vi "ConfigWindow.vi"(8 "error in":errorcluster) -> (0 "error out":errorcluster, 3 "COM Bluegiga out":refnum<visa-resource-name>, 4 "Connection Status":T1={"MAC Address"="", "cnx handle"=0, "cnx flags"=0, "Address Type"=0, "Connection Interval (ms)"=125, "Timeout(ms)"=125, "Latency"=125, "bonding handle"=0} {"Address Type" items=["Public", "Random"]})   [LabVIEW 2015]
uses:
  <vilib>/BLE/type_def/connection_status_bundle.ctl
  <vilib>/BLE/type_def/address_type.ctl
panel:
  in  "Save to Database":bool=TRUE
  in  "CONNECT":bool caption="Power"
  out "Choosen adress":string caption="String"
  out "Tab":string[][](array[string]) caption="Donge info"
  in  "SCAN":bool caption="Search"
  out "Donge info":string caption="String"
  in  "BLE Dongle VISA":refnum<visa-resource-name>
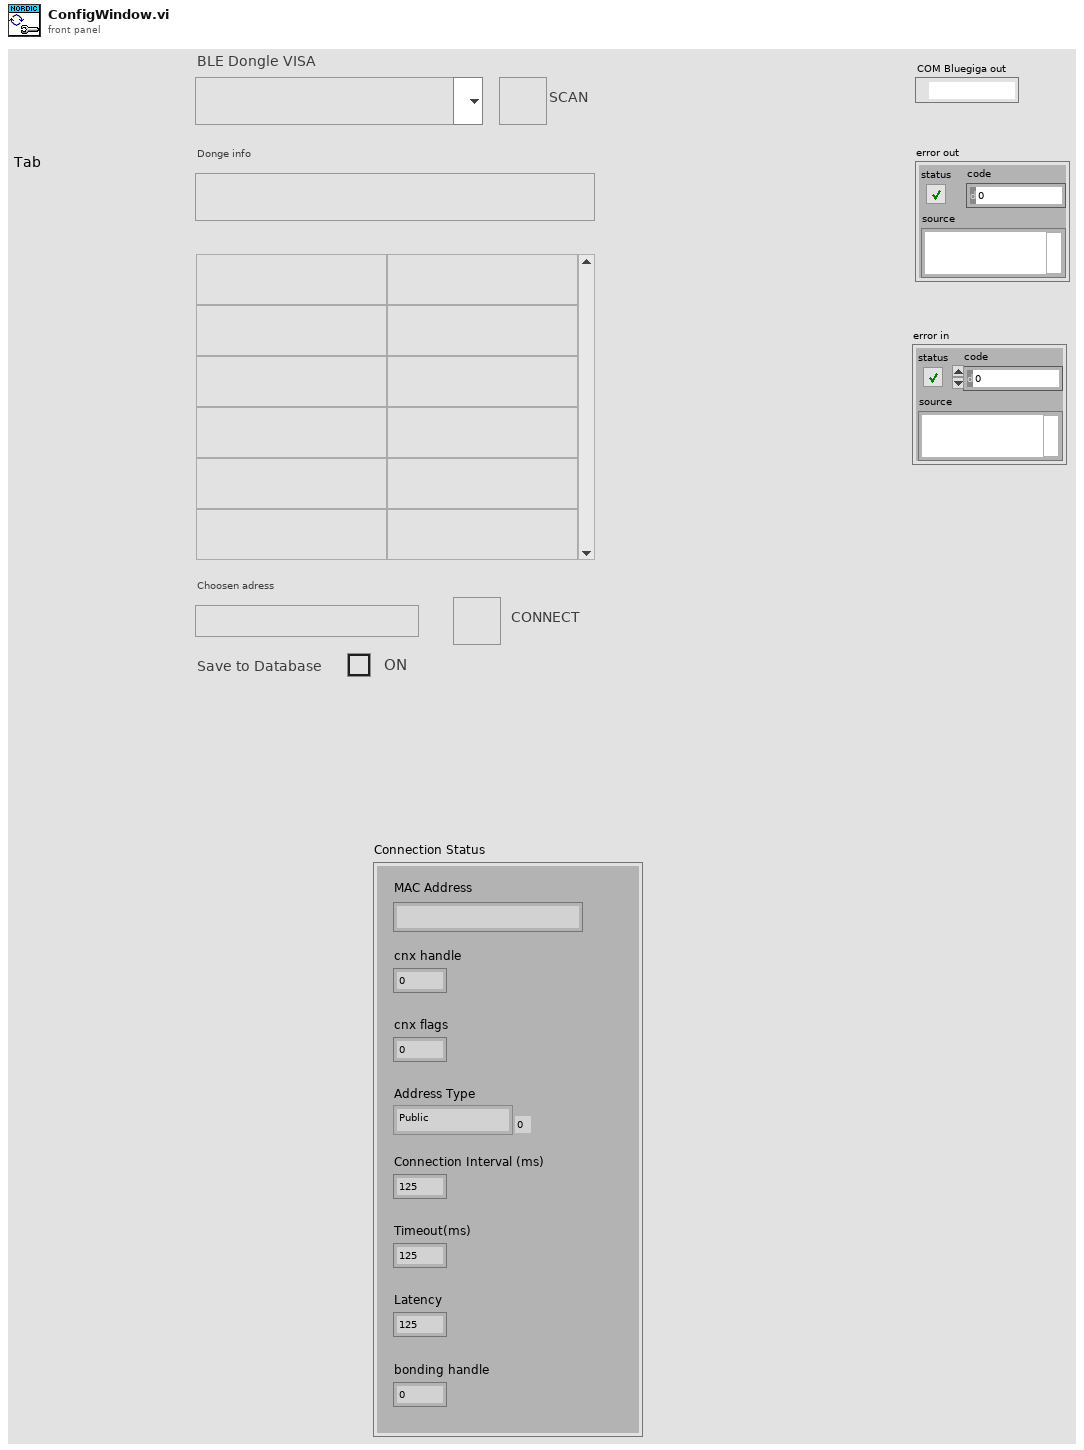
[diagram p1: front panel]
types:
  T1 = typedef "connection_status_bundle.ctl" = cluster{"MAC Address":string, "cnx handle":u8, "cnx flags":u8, "Address Type":T2, "Connection Interval (ms)":u16, "Timeout(ms)":u16, "Latency":u16, "bonding handle":u8}
  T2 = typedef "address_type.ctl" = u8
  T3 = enum8{"Enabled", "Disabled", "Disabled and Grayed Out"}
  T4 = typedef "LVPoint32TypeDef.ctl" = cluster{"Horizontal":i32, "Vertical":i32}
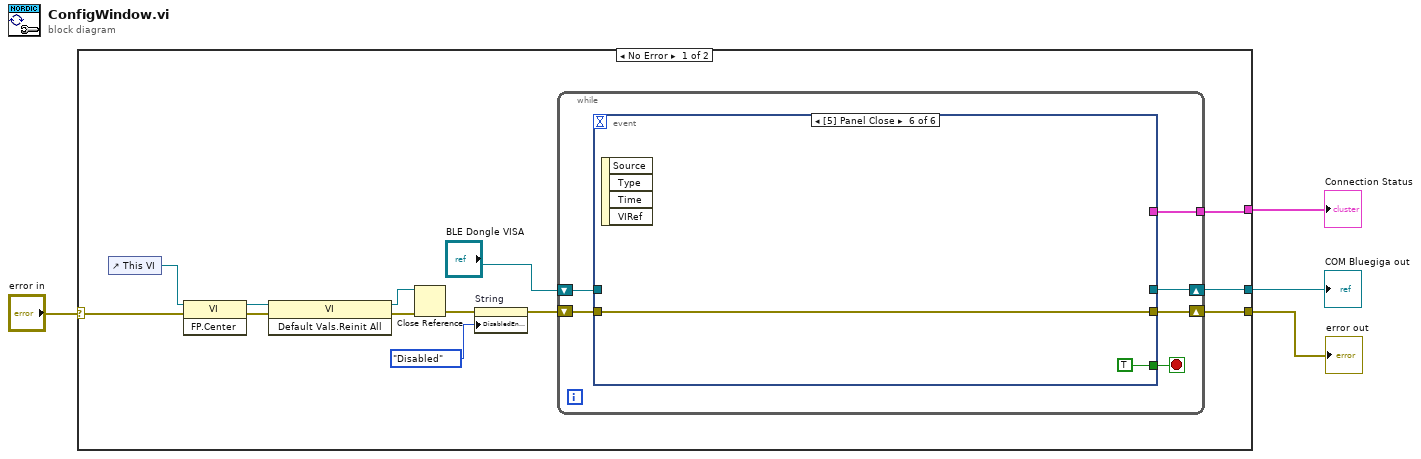
[diagram p0: block diagram]
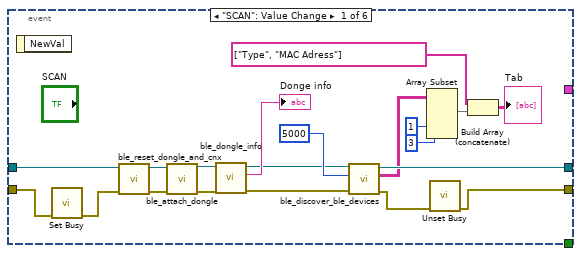
[diagram p2: hidden frame]
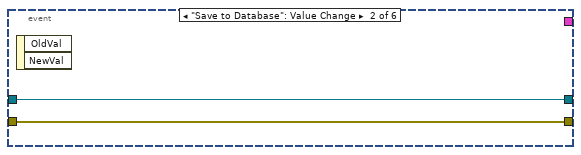
[diagram p3: hidden frame]
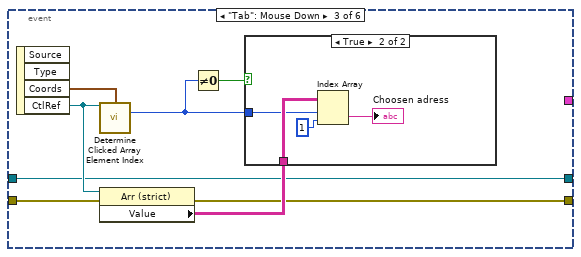
[diagram p4: hidden frame]
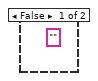
[diagram p5: hidden frame]
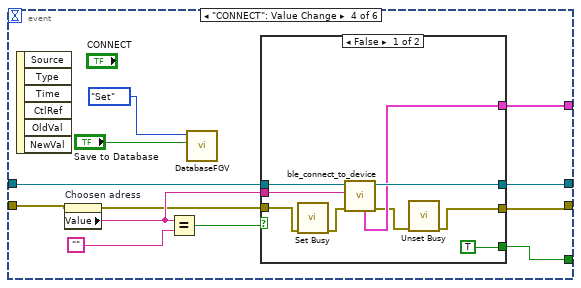
[diagram p6: hidden frame]
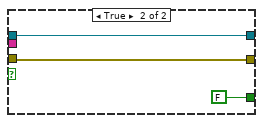
[diagram p7: hidden frame]
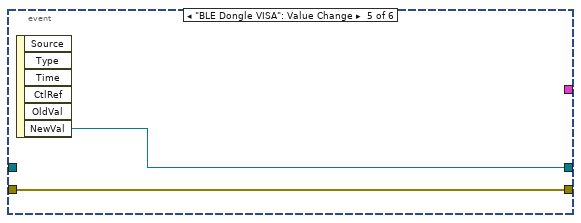
[diagram p8: hidden frame]
diagram:
  n1 = case shown="No Error" "error in" {
    selector: "error in" -> [w9 w86]
    tunnel: [w15 _] -> w4
    tunnel: [w14 w86] -> w3
    tunnel: [w5 _] -> w1
    frame No Error {
      n2 = control-ref of="This VI"() -> (w8:refnum<vi>)
      n3 = invoke class="VI" method="FP.Center"(reference=w8, error in=w9) -> (reference out=w7:refnum<vi>, error out=w6:errorcluster)  [unwired: 1 in, 1 out]
      n4 = invoke class="VI" method="Default Vals.Reinit All"(reference=w7, error in=w6) -> (reference out=w11:refnum<vi>, error out=w12:errorcluster)  [unwired: 1 in, 1 out]
      n5 = Close Reference(reference=w11, error in (no error)=w12) -> (error out=w10:errorcluster)
      n6 = property on="String" class="Str"(error in=w10, "DisabledEnum"=T3."Disabled" ("Disabled")) -> (error out=w13:errorcluster)  [unwired: 1 in, 1 out]
      n7 = while {
        shift-right: [w20] -> w14
        shift-left: w13 -> [w22]
        shift-right: [w19] -> w15
        shift-left: "BLE Dongle VISA" -> [w23]
        tunnel: [w18] -> w5
        stop <- w21 stop-if-true
        n8 = event shown="[5] Panel Close" {
          selector: _ -> [_ _ _ _ _ _]
          dyn-events: _ -> [_ _ _ _ _ _]
          timeout: _ -> [_ _ _ _ _ _]
          tunnel: w23 -> [w40 w44 w46 w63 _ _]
          tunnel: w22 -> [w37 w45 w51 w66 w82 w84]
          tunnel: [w31 w44 w46 w61 w83 _] -> w19
          tunnel: [_ _ _ w67 _ TRUE] -> w21
          tunnel: [w27 w45 w49 w62 w82 w84] -> w20
          tunnel: [_ _ _ w60 _ _] -> w18
          event "SCAN": Value Change {
            n9 = event-data() -> ()  [unwired: 1 in, 1 out]
            n10 = call <vilib>:"Set Busy.vi"("error in (no error)"=w37) -> ("error out"=w36:errorcluster)  [unwired: 9 in, 1 out]
            n11 = call <vilib>:"ble_reset_dongle_and_cnx.vi"("error in (no error)"=w36, "COM Bluegiga in"=w40) -> ("error out"=w39:errorcluster, "COM Bluegiga out"=w42:refnum<visa-resource-name>)  [unwired: 8 in]
            n12 = call <vilib>:"ble_attach_dongle.vi"("error in (no error)"=w39, "COM Bluegiga in"=w42) -> ("error out"=w38:errorcluster, "COM Bluegiga out"=w41:refnum<visa-resource-name>)  [unwired: 8 in]
            n13 = call <vilib>:"ble_dongle_info.vi"("error in (no error)"=w38, "COM Bluegiga in"=w41) -> ("error out"=w34:errorcluster, "info"=→"Donge info":string, "COM Bluegiga out"=w33:refnum<visa-resource-name>)  [unwired: 7 in]
            n14 = call <vilib>:"ble_discover_ble_devices.vi"("error in (no error)"=w34, "Scan Duration (10000ms)"=u32 5000, "COM Bluegiga in"=w33) -> ("error out"=w32:errorcluster, "Devices"=w30:string[][], "COM Bluegiga out"=w31:refnum<visa-resource-name>)  [unwired: 6 in]
            n15 = Array Subset(array=w30, index (col)=1 ("index"), length (col)=3 ("index")) -> (w25:string[][])  [unwired: 2 in]
            n16 = call <vilib>:"Unset Busy.vi"("error in (no error)"=w32) -> ("error out"=w27:errorcluster)  [unwired: 10 in]
            n17 = Build Array (concatenate)(string[] ["Type", "MAC Adress"] ("element"), w25) -> (→"Tab":string[][])
          }
          event "Save to Database": Value Change {
            n18 = event-data() -> ()  [unwired: 1 in, 2 out]
          }
          event "Tab": Mouse Down {
            n19 = event-data() -> ("Coords"=w52:T4, "CtlRef"=w50:refnum<vi>)  [unwired: 1 in, 2 out]
            n20 = call "Determine Clicked Array Element Index.vi"("reference"=w50, "Coords of Click"=w52) -> ("Clicked Row"=w47:i32)  [unwired: 8 in, 5 out]
            n21 = property class="Arr (strict)"(reference=w50, error in=w51) -> (error out=w49:errorcluster, "Value"=w53:string[][])  [unwired: 1 out]
            n22 = Not Equal To 0?(x=w47) -> (x != 0?=w48:bool)
            n23 = case shown="True" w48 {
              tunnel: w53 -> [_ w57]
              tunnel: w47 -> [_ w55]
              frame False {
                (unwired) "" ("String")
              }
              frame True {
                n24 = Index Array(array=w57, index (row)=w55, index (col)=1 ("disabled index (col)")) -> (element=→"Choosen adress":string)
              }
            }
          }
          event "CONNECT": Value Change {
            n25 = event-data() -> ()  [unwired: 1 in, 6 out]
            n26 = property on="Choosen adress" class="Str"(error in=w66) -> (error out=w64:errorcluster, "Value"=w65:string)  [unwired: 1 in, 1 out]
            n27 = Equal?(x=w65, y="") -> (x = y?=w68:bool)
            n28 = call "DatabaseFGV.vi"("Set"="Save to Database", "State"=enum16{"Get", "Set"}."Set") -> ()  [unwired: 9 in, 1 out]
            n29 = case shown="False" w68 {
              tunnel: [TRUE FALSE] -> w67
              tunnel: w65 -> [w76 _]
              tunnel: w64 -> [w73 w79]
              tunnel: w63 -> [w77 w80]
              tunnel: [w70 w79] -> w62
              tunnel: [w75 w80] -> w61
              tunnel: [w74 _] -> w60
              frame False {
                n30 = call <vilib>:"Set Busy.vi"("error in (no error)"=w73) -> ("error out"=w72:errorcluster)  [unwired: 9 in, 1 out]
                n31 = call <vilib>:"ble_connect_to_device.vi"("error in (no error)"=w72, "MAC Address"=w76, "COM Bluegiga in"=w77) -> ("error out"=w71:errorcluster, "COM Bluegiga out"=w75:refnum<visa-resource-name>, "Connection Status"=w74:T1)  [unwired: 6 in]
                n32 = call <vilib>:"Unset Busy.vi"("error in (no error)"=w71) -> ("error out"=w70:errorcluster)  [unwired: 10 in]
              }
              frame True {
              }
            }
          }
          event "BLE Dongle VISA": Value Change {
            n33 = event-data() -> ("NewVal"=w83:refnum<visa-resource-name>)  [unwired: 1 in, 5 out]
          }
          event Panel Close {
            n34 = event-data() -> ()  [unwired: 1 in, 4 out]
          }
        }
      }
    }
    frame Error {
    }
  }
  "COM Bluegiga out" <- w4
  "error out" <- w3
  "Connection Status" <- w1
